vi "Write Counter New Setpoint.vi"(8 "error in":errorcluster, 10 "New Setpoint Value":u16, 11 "MB_TCP session in":refnum<class "MB_Master_TCP.lvclass">) -> (0 "error out":errorcluster, 2 "Counter New Setpoint":u16, 3 "MB session out":refnum<class "MB_Master_TCP.lvclass">)   [LabVIEW 2024, in "Bronkhorst Flexi-Flow ModbusTCP API.lvlib"]
uses:
  Bronkhorst Flexi-Flow ModbusTCP API.lvlib
  <vilib>/Plasmionique/MB Master/MB_Master_TCP/MB_Master_TCP.lvclass
  PDU Address Float 32-bit Params--ring.ctl
  Write Unsigned Int Register.vi
  Read Unsigned Int Register.vi
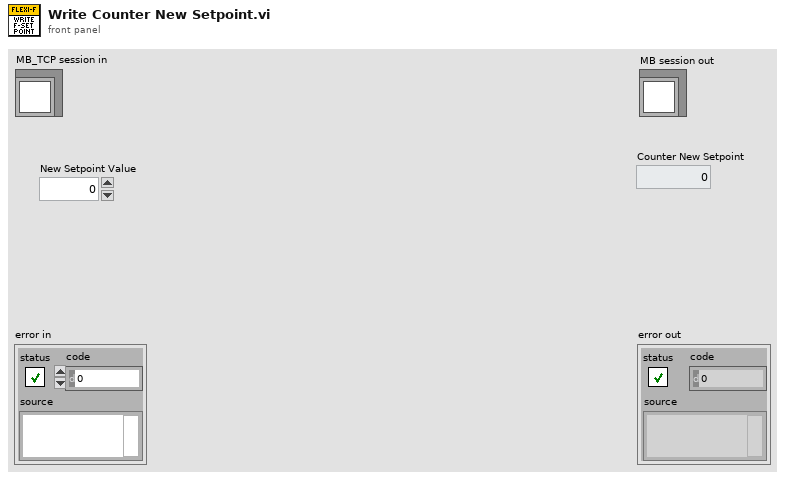
[diagram p1: front panel]
types:
  T1 = typedef "Bronkhorst Flexi-Flow ModbusTCP API.lvlib/PDU Address Float 32-bit Params--ring.ctl" = u16
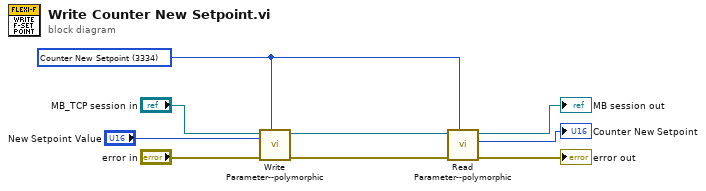
[diagram p0: block diagram]
diagram:
  w3 = T1 3334 items=["Counter New Setpoint"=3334, "FSetpoint (Channel F)"=41240, "Fmeasure (Channel F)"=41216, "FSetpoint (Channel P1)"=41496, "Fmeasure (Channel P1)"=41472, "FSetpoint (Channel P2)"=41752, "Fmeasure (Channel P2)"=41728, "Capacity 0%"=41392, "Counter limit (Float)"=59416, "Inlet Pressure"=61801, "Outlet Pressure"=61809, "PID-Kp"=62120, "PID-Ti"=62128, "PID-Td"=62136, "Dynamic display factor"=62728, "Static display factor"=62736, "Exponential smoothing"=62752] ("PDU Address 32-bit Float")
  n1 = call-poly "Write Parameter--polymorphic.vi"("PDU Address (U-Int16)"=w3, "error in"="error in", "Value"="New Setpoint Value", "MB_TCP session in"="MB_TCP session in") -> ("error out"=w5:errorcluster, "MB session out"=w7:refnum<class "MB_Master_TCP.lvclass">)  [unwired: 6 in]
  n2 = call-poly "Read Parameter--polymorphic.vi"("PDU Address (U-Int16)"=w3, "error in"=w5, "MB_TCP session in"=w7) -> ("error out"=→"error out":errorcluster, "Value"=→"Counter New Setpoint":u16, "MB session out"=→"MB session out":refnum<class "MB_Master_TCP.lvclass">)  [unwired: 6 in]
